vi "WS1050 16 DUT VSA-CV Sweep HD_Cycling_Ver1.1.vi"() -> ()   [LabVIEW 2012]
uses:
  WS_VCAP Driver 024/Source/WSVCAP Shell/Type Defs/WSVCAP SHL I2C DUT Mask Mode Enum.ctl
  <vilib>/Utility/file.llb/Read From Spreadsheet File (DBL).vi
panel:
  out "VISA resource name out":refnum<visa-resource-name>="GPIB0::3::INSTR"
  out "date string":string="5/19/2014"
  out "PS1 Out":refnum<visa-resource-name>
  out "Ke2000 Out":refnum<visa-resource-name>="GPIB0::9::INSTR"
  in  "Tab Control":enum32{"Inst Control", "Data Output", "Graphs"}(tab)
  in  "Bank to Stress":u16(ring) items=["All OFF", "All ON", "Bank_C1", "Bank_C2", "Bank_C3"]
  out "AD7747 Values":string[][](table)
  in  "Lot#":string="4NEMB"
  in  "Wafer#":string="20-EB"
  in  "File Name":string="HD_4NEMB_25_EB_65C_44V_100DC_BRD2_150916_1"
  in  "TMN DC\\CAP Data Log File Path":path=path "C:/WS1050 16 DUT Data"
  in  "SN":string[](array[string])=["1", "2", "3", "4", "5", "6", "7", "8", "9", "10", "11", "12", "13", "14", "15", "16"]
  in  "Test Program":string="WS1050 16 DUT VSA_CV Sweep HD_Cycling Ver1.2"
  out "Current Date":string="8/28/2014"
  out "Current Time":string="0950"
  in  "Start Date":string="4/24/2014"
  in  "Start Time":string="1542"
  in  "Comment":string="VSA CV Sweep"
  in  "OK Button":bool
  in  "Calibration":bool
  in  "Control Setting":bool
  in  "CP Setting":i32(ring) items=["CP OFF", "CP ON", "CP 35V", "CP 40V", "CP 44V", "CP 50V", "DVA OFF", "DVA ON", "Reg1 ON", "Reg1 OFF", "Reg2 ON", "Reg2 OFF", "Reg3 ON", "Reg3 OFF"]
  in  "VDD(V)":dbl=3.3 format="%.3g"
  in  "SPI Clock Rate (Hz)":dbl=1000000.0 caption="Meas Speed" format="%.1p Hz"
  out "AR  Measurent(Hz)":dbl
  in  "PS1 Source":refnum<visa-resource-name>="GPIB0::5::INSTR"
  in  "Ke2000":refnum<visa-resource-name>="GPIB0::9::INSTR"
  out "Simulate FPGA":bool
  out "Online":bool
  in  "Ke2400":refnum<visa-resource-name>="GPIB0::3::INSTR"
  in  "Initialize AD7747":bool
  in  "DUT Mask Mode":T1=enum."All"
  in  "RFFE Slave Address":u8=7 caption="Slave Address" format="0x%02x"
  out "Activity Log":string="05/19/2014 -- 12:24:35.853::WSVCAP::APP::Application Started\n05/19/2014 -- 12:24:37.606::WSVCAP::WSVCAP SHL::WR I2C-REG:0x0A;MASK:0xFFFFFFFFFFFF;C1 DATA:22:22:22:22:22:22:22:22:22:22:22:22:22:22:22:22;C2 DATA:22:22:22:22:22:22:22:22:22:22:22:22:22:22:22:22;C3 DATA:22:22:22:22:22:22:22:22:22:22:22:22:22:22:22:22\r\n05/19/2014 -- 12:24:37.773::WSVCAP::WSVCAP SHL::WR I2C-ST:0,0,4,1\r\n05/19/2014 -- 12:24:37.903::WSVCAP::WSVCAP SHL::RD I2C-BYTES:4;ADD:0x00;MASK:0xFFFFFFFFFFFF\r\n05/19/2014 -- 12:24:38.045::WSVCAP::WSVCAP SHL::RD I2C:C1 DATA:2:2:2:2:2:2:2:2:2:2:2:2:2:2:2:2|A7:A9:AA:82:82:7F:82:81:82:81:83:82:81:82:82:81|46:36:BB:88:44:A3:E9:2B:32:20:ED:25:BB:3D:68:B|2C:6A:EB:A7:22:56:FE:CC:36:82:D7:B0:3B:48:F9:CC;C2 DATA:2:2:2:2:2:2:2:2:2:2:2:2:2:2:2:2|94:94:94:80:80:80:80:80:81:7E:7E:81:80:7E:80:80|47:33:15:82:62:B:E8:1C:D7:C3:7D:41:7C:B7:4C:2A|C4:B4:AE:8:1E:D1:4E:37:11:C0:6F:63:42:9D:63:B5;C3 DATA:2:2:2:2:2:2:2:2:2:2:2:2:2:2:2:2|95:95:95:81:81:7E:81:80:84:7D:80:83:81:7E:7F:80|AB:C4:14:B5:7B:52:DF:C9:79:5D:5F:30:99:31:1E:F4|6E:5C:F7:A8:C3:EB:7B:EF:33:92:89:77:4D:67:75:DD;STATUS:0:0:4:0\r\n05/19/2014 -- 12:24:38.046::WSVCAP::WSVCAP SHL::WR I2C-REG:0x0A;MASK:0xFFFFFFFFFFFF;C1 DATA:22:22:22:22:22:22:22:22:22:22:22:22:22:22:22:22;C2 DATA:22:22:22:22:22:22:22:22:22:22:22:22:22:22:22:22;C3 DATA:22:22:22:22:22:22:22:22:22:22:22:22:22:22:22:22\r\n05/19/2014 -- 12:24:38.089::WSVCAP::WSVCAP SHL::WR I2C-ST:0,0,4,1\r\n05/19/2014 -- 12:24:38.219::WSVCAP::WSVCAP SHL::RD I2C-BYTES:4;ADD:0x00;MASK:0xFFFFFFFFFFFF\r\n05/19/2014 -- 12:24:38.362::WSVCAP::WSVCAP SHL::RD I2C:C1 DATA:2:2:2:2:2:2:2:2:2:2:2:2:2:2:2:2|A7:AB:AA:82:82:82:83:83:82:82:82:82:7F:82:82:81|4B:32:96:83:3E:61:43:17:25:62:AB:4D:A2:40:2E:5|3C:76:2B:B4:EE:E4:A9:1A:AA:A:26:C7:21:2E:87:5B;C2 DATA:2:2:2:2:2:2:2:2:2:2:2:2:2:2:2:2|94:94:94:80:80:80:80:80:80:7F:80:81:80:80:7F:80|4A:32:19:7D:19:6C:79:46:61:7F:4B:B8:A5:30:F3:14|B4:70:A:8C:9C:DC:43:FA:1E:A:C6:21:A:A9:13:F3;C3 DATA:2:2:2:2:2:2:2:2:2:2:2:2:2:2:2:2|95:97:94:81:80:81:82:81:80:7E:81:84:7F:81:80:80|B2:32:D0:A7:9E:4C:AB:D4:EE:D9:F0:82:B7:91:7:FF|C1:91:B6:3D:D8:E:1B:4F:9F:6A:F1:6C:E7:3F:7:BA;STATUS:0:0:4:0\r\n05/19/2014 -- 12:24:38.364::WSVCAP::WSVCAP SHL::WR I2C-REG:0x0A;MASK:0xFFFFFFFFFFFF;C1 DATA:22:22:22:22:22:22:22:22:22:22:22:22:22:22:22:22;C2 DATA:22:22:22:22:22:22:22:22:22:22:22:22:22:22:22:22;C3 DATA:22:22:22:22:22:22:22:22:22:22:22:22:22:22:22:22\r\n05/19/2014 -- 12:24:38.406::WSVCAP::WSVCAP SHL::WR I2C-ST:0,0,4,1\r\n05/19/2014 -- 12:24:38.536::WSVCAP::WSVCAP SHL::RD I2C-BYTES:4;ADD:0x00;MASK:0xFFFFFFFFFFFF\r\n05/19/2014 -- 12:24:38.678::WSVCAP::WSVCAP SHL::RD I2C:C1 DATA:2:2:2:2:2:2:2:2:2:2:2:2:2:2:2:2|A7:A9:AB:82:82:81:82:82:82:82:82:82:82:82:82:81|46:71:4C:87:43:3D:7F:FC:25:4F:8E:54:97:3E:60:8C|AA:F4:1F:B5:CE:43:1F:36:9:87:9C:78:86:5:B6:8E;C2 DATA:2:2:2:2:2:2:2:2:2:2:2:2:2:2:2:2|94:94:94:80:7F:7F:80:80:80:80:80:81:80:80:80:80|49:36:18:7D:6E:C5:E4:3C:81:2E:41:D3:75:71:E3:72|E8:D3:E6:D1:E0:48:AE:D4:54:D:E8:8E:B4:41:68:4;C3 DATA:2:2:2:2:2:2:2:2:2:2:2:2:2:2:2:2|95:95:95:81:7F:7F:81:81:81:81:81:84:81:81:82:81|B3:F5:90:AB:82:69:7B:93:D0:77:E8:D5:E8:8C:84:E8|B9:AC:EE:2B:B6:71:8F:4A:74:31:56:BB:8A:B7:A0:C8;STATUS:0:0:4:0\r\n05/19/2014 -- 12:24:38.681::WSVCAP::WSVCAP SHL::WR I2C-REG:0x0A;MASK:0xFFFFFFFFFFFF;C1 DATA:22:22:22:22:22:22:22:22:22:22:22:22:22:22:22:22;C2 DATA:22:22:22:22:22:22:22:22:22:22:22:22:22:22:22:22;C3 DATA:22:22:22:22:22:22:22:22:22:22:22:22:22:22:22:22\r\n05/19/2014 -- 12:24:38.723::WSVCAP::WSVCAP SHL::WR I2C-ST:0,0,4,1\r\n05/19/2014 -- 12:24:38.854::WSVCAP::WSVCAP SHL::RD I2C-BYTES:4;ADD:0x00;MASK:0xFFFFFFFFFFFF\r\n05/19/2014 -- 12:24:38.996::WSVCAP::WSVCAP SHL::RD I2C:C1 DATA:2:2:2:2:2:2:2:2:2:2:2:2:2:2:2:2|A7:A9:AA:82:82:7F:83:81:82:81:84:82:7F:82:7F:82|43:FB:E:7F:3C:AD:35:35:26:A2:6C:21:4B:3D:8:6|63:9A:E1:F3:95:32:91:42:90:3C:78:1F:5C:D7:5F:D8;C2 DATA:2:2:2:2:2:2:2:2:2:2:2:2:2:2:2:2|94:94:94:80:80:80:80:80:81:80:7E:81:80:7E:7F:80|48:36:18:7F:5E:3D:69:83:DE:AE:A1:9E:31:AE:BB:96|15:A0:44:17:13:FD:CC:C8:6D:B2:EF:A7:C:C7:3B:F;C3 DATA:2:2:2:2:2:2:2:2:2:2:2:2:2:2:2:2|95:96:94:81:81:7E:82:80:84:80:80:84:7F:7E:7D:82|AD:3B:6D:A9:7C:57:9D:F5:7A:96:23:5C:36:2D:ED:5A|CD:46:DB:3B:C7:BD:70:60:33:B8:B:F7:63:A:51:4D;STATUS:0:0:4:0\r\n05/19/2014 -- 12:24:38.998::WSVCAP::WSVCAP SHL::WR I2C-REG:0x0A;MASK:0xFFFFFFFFFFFF;C1 DATA:22:22:22:22:22:22:22:22:22:22:22:22:22:22:22:22;C2 DATA:22:22:22:22:22:22:22:22:22:22:22:22:22:22:22:22;C3 DATA:22:22:22:22:22:22:22:22:22:22:22:22:22:22:22:22\r\n05/19/2014 -- 12:24:39.040::WSVCAP::WSVCAP SHL::WR I2C-ST:0,0,4,1\r\n05/19/2014 -- 12:24:39.170::WSVCAP::WSVCAP SHL::RD I2C-BYTES:4;ADD:0x00;MASK:0xFFFFFFFFFFFF\r\n05/19/2014 -- 12:24:39.311::WSVCAP::WSVCAP SHL::RD I2C:C1 DATA:2:2:2:2:2:2:2:2:2:2:2:2:2:2:2:2|A7:AA:AB:82:82:81:82:81:82:81:82:82:82:82:7F:82|44:F1:90:87:45:44:C8:2C:2C:F1:FC:1B:94:3B:3C:75|4A:49:95:19:99:73:64:3:23:24:F3:A2:5E:7F:C4:B6;C2 DATA:2:2:2:2:2:2:2:2:2:2:2:2:2:2:2:2|94:94:94:80:80:80:80:7F:80:80:7E:80:80:7E:7F:80|4C:36:17:7D:A8:9F:DE:C7:53:6D:8A:F4:41:A5:C6:E0|90:2E:24:C:D9:22:E4:76:3B:40:1D:53:33:B1:3E:4D;C3 DATA:2:2:2:2:2:2:2:2:2:2:2:2:2:2:2:2|95:97:95:81:81:7F:81:80:80:81:7F:82:81:7E:7D:82|AE:2B:A7:AB:CC:CD:A4:38:FD:17:80:F2:92:2D:45:C4|76:E5:D:B9:AD:B5:BA:8D:28:32:9E:42:B7:20:4A:D9;STATUS:0:0:4:0\r\n05/19/2014 -- 12:24:39.313::WSVCAP::WSVCAP SHL::WR I2C-REG:0x0A;MASK:0xFFFFFFFFFFFF;C1 DATA:22:22:22:22:22:22:22:22:22:22:22:22:22:22:22:22;C2 DATA:22:22:22:22:22:22:22:22:22:22:22:22:22:22:22:22;C3 DATA:22:22:22:22:22:22:22:22:22:22:22:22:22:22:22:22\r\n05/19/2014 -- 12:24:39.355::WSVCAP::WSVCAP SHL::WR I2C-ST:0,0,4,1\r\n05/19/2014 -- 12:24:39.486::WSVCAP::WSVCAP SHL::RD I2C-BYTES:4;ADD:0x00;MASK:0xFFFFFFFFFFFF\r\n05/19/2014 -- 12:24:39.628::WSVCAP::WSVCAP SHL::RD I2C:C1 DATA:2:2:2:2:2:2:2:2:2:2:2:2:2:2:2:2|A7:A9:AA:82:82:82:83:82:82:82:82:82:7F:82:7F:82|47:18:E4:87:3E:E7:6:65:25:92:37:38:A8:3E:89:85|7C:A7:7:2B:A3:7A:EC:EF:89:ED:F4:D3:D8:BC:3A:F5;C2 DATA:2:2:2:2:2:2:2:2:2:2:2:2:2:2:2:2|94:94:94:80:7F:80:80:7F:81:80:7E:80:80:80:81:80|49:37:17:80:76:25:6A:F8:DF:55:97:4D:B8:5B:2B:B1|13:E3:9A:3E:1A:2D:4F:B6:DB:E9:61:FA:8B:D6:9:CC;C3 DATA:2:2:2:2:2:2:2:2:2:2:2:2:2:2:2:2|95:95:95:81:7F:80:82:81:84:80:7F:81:80:81:7F:82|AF:93:3B:AF:5B:11:82:E4:7E:C3:2D:72:9:96:D9:A|DB:96:F2:10:5F:64:9A:C6:98:12:27:7D:10:D3:20:D9;STATUS:0:0:4:0\r\n05/19/2014 -- 12:24:40.132::WSVCAP::WSVCAP SHL::CLOSE\r\n"
  in  "C1 Cap DAC":u8=128 caption="B Data In" format="0x%02x"
  in  "C2 Cap DAC":u8=128 caption="B Data In" format="0x%02x"
  in  "C3 Cap DAC":u8=128 caption="B Data In" format="0x%02x"
  out "IDD Brd(uA)":string
  in  "VSA_IDD(A)":dbl=0.1
  in  "Stress Voltage(V)":dbl=10.0
  in  "CP to HD/Cycle":i32(ring)=4 items=["CP HDC 35V", "CP HDC 40.25V", "CP HDC 27.5V", "CP HDC 30.5V", "CP HDC 44V", "CP HDC 50V"]
  in  "Reset PS":bool
  out "STATUS":string="Idle...."
  in  "stop":bool
  out "C1 Min_T0":string[](array[string])
  out "CAP_Value(pF)":string[][](array[string])
  out "C3 Min_T0":string[](array[string])
  out "C2 Min_T0":string[](array[string])
  in  "Abort":bool
  out "error out 2":errorcluster
  in  "Set HD Time \nto Complete(Min)":u64=8100
  out "HD Time\nCompleted(Min)":u64
  out "Verify Test Condition":string[](array[string])
  out "CMin+VCAP":string[][](table)
  out "Previous Time":string="12:20:26 PM"
  out "Running Loops":i32=1
  out "Verify Drivers to Stress":string[](array[string])
  out "Delta CAP_T0(pF)":dbl[][](array[numeric])
  out "Delta CAP_Tc(pF)":dbl[][](array[numeric])
  in  "error in (no error)":errorcluster
  out "error out":errorcluster
  out "CP_IDD(uA)":string
  # "Company:  WiSpry Inc 20 Fairbanks \nSte 198 Irvine CA 92618\n\nAuthor:  Andy V Tran\nCreated:  11/23/2015\nLabVIEW 2012 Pro\nTP:  WS1050 16 DUT VSA_CV Sweep HD_Cycling Ver1.1\nFPGA Version: WS_VCAP Driver 024"
  # "Note:  Ver1.0 is a original version.\n\n1.  Two look up tables, \n      a.  1st is for Stress\n      b.  2nd is for Voltage sweep\n\nVer1.1\n\n1.  No Voltage to CAP Head for initial read point\n\nSet up and Test Sequences:\n\n1.  Calibration with Empty Sockets\n2.  Load Parts\n3.  Set condition to stress (CP Voltage, Drivers to Stress, CP to stress...)\n4.  Set Date/Time to start stressing\n5.  Set TTF to stop stressing (default = 135 hrs)"
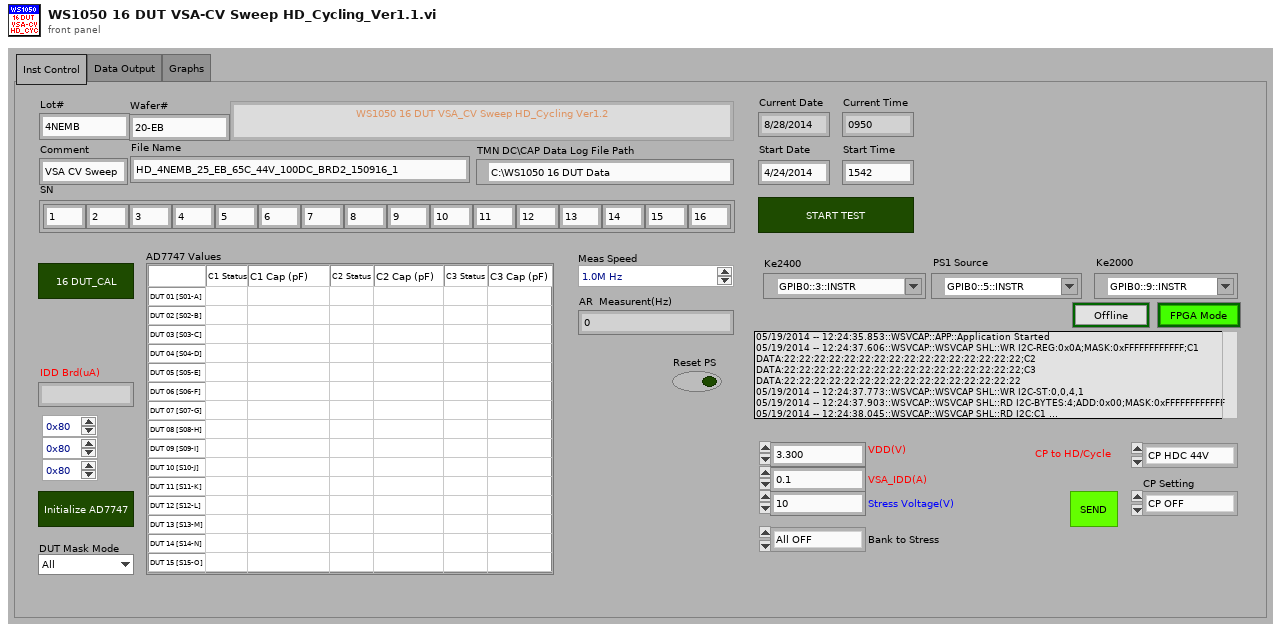
[diagram p1: front panel]
types:
  T1 = typedef "WSVCAP SHL I2C DUT Mask Mode Enum.ctl" = enum16{"Custom", "C1", "C2", "C3", "All"}
  T2 = typedef "WSVCAP SHL Core System Cluster.ctl" = cluster{"Settings":T3, "FPGA Resource":tag, "Online":bool, "I2C Wait Ticks":u32, "SPI Wait Ticks":u32, "RFFE Wait Ticks":u32}
  T3 = typedef "WSVCAP SHL I2C Settings Cluster.ctl" = cluster{"FPGA Resource Name":string, "I2C Slave Address":u8, "I2C Clock Rate (Hz)":dbl, "SPI Clock Rate (Hz)":dbl, "RFFE Slave Address":u8, "RFFE Clock Rate (Hz)":dbl, "Simulate FPGA":bool, "C1 Cap DAC Default":u8, "C2 Cap DAC Default":u8, "C3 Cap DAC Default":u8}
  T4 = enum16{"Idle...", "Voltage 1", "Voltage 2", "Voltage 3"}[]
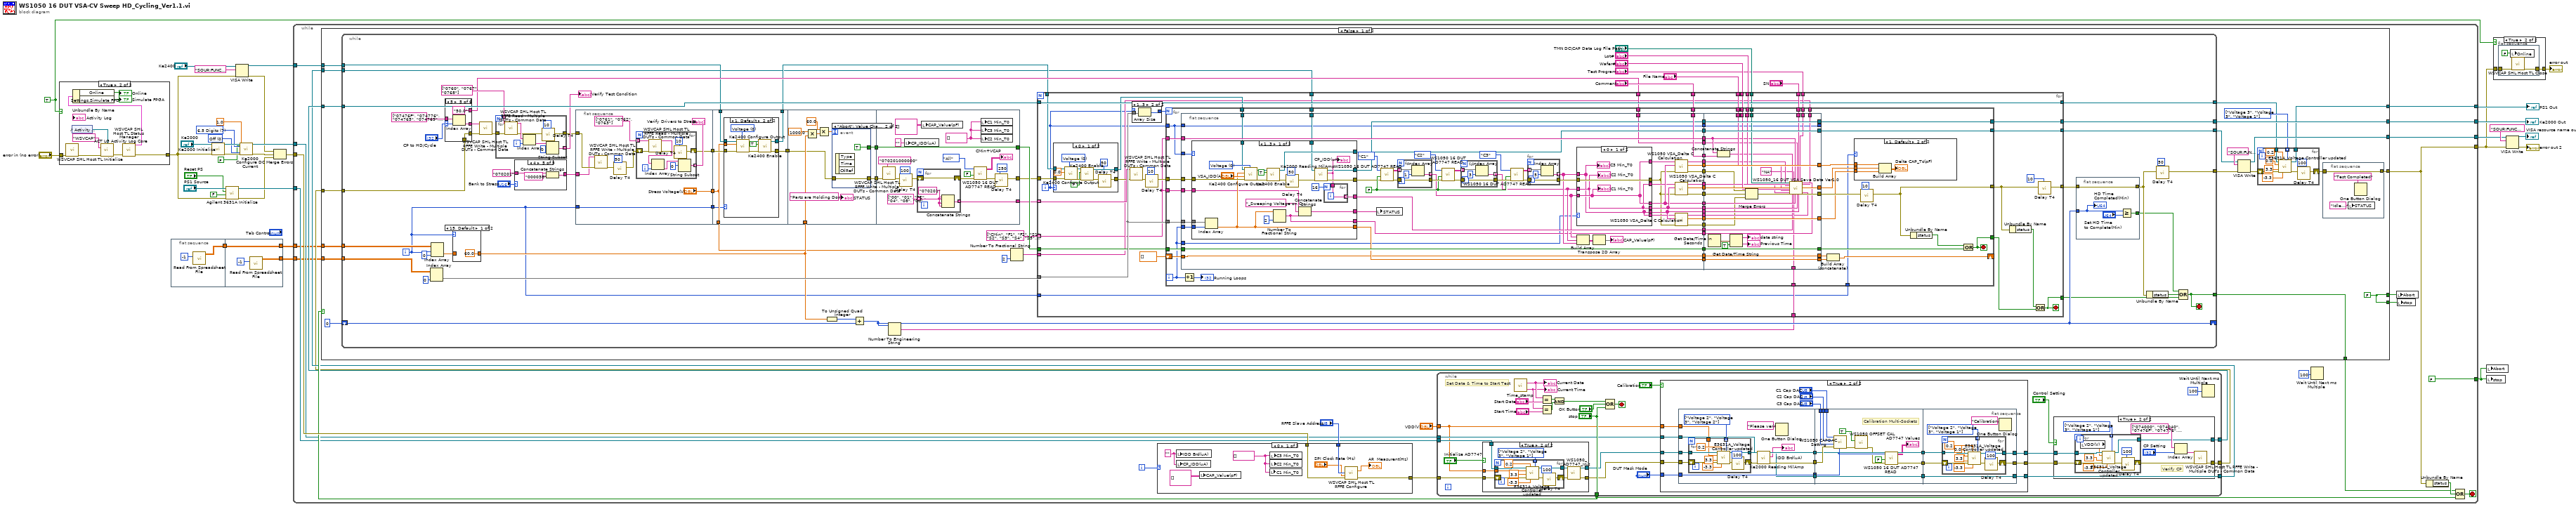
[diagram p0: block diagram]
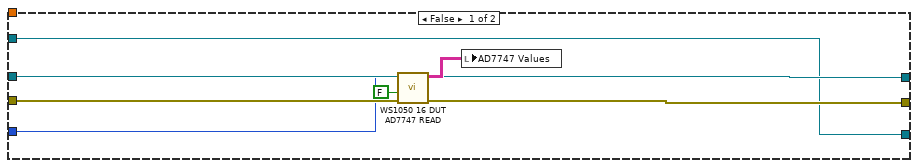
[diagram p7: hidden frame]
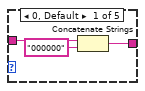
[diagram p8: hidden frame]
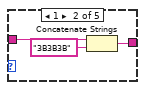
[diagram p9: hidden frame]
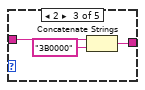
[diagram p10: hidden frame]
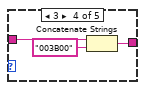
[diagram p11: hidden frame]
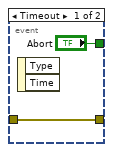
[diagram p14: hidden frame]
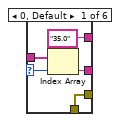
[diagram p15: hidden frame]
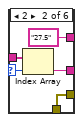
[diagram p16: hidden frame]
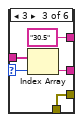
[diagram p17: hidden frame]
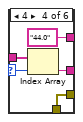
[diagram p18: hidden frame]
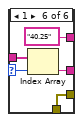
[diagram p19: hidden frame]
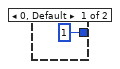
[diagram p20: hidden frame]
diagram:
  w21 = TRUE
  w27 = u16 0 items=["Off", "Moving Filter", "Repeating Filter"] ("Digital Filter (0: Off)")
  w28 = u16 7 items=["3.5 Digits"=4, "4.5 Digits"=5, "5.5 Digits"=6, "6.5 Digits"=7] ("Resolution (7: 6.5 digits)")
  n1 = case shown="True" w21 {
    tunnel: "error in (no error)" -> [w35 w36]
    tunnel: [w35 w43] -> w10
    frame False {
    }
    frame True {
      n2 = call "WSVCAP SHL Host TL Initialize.vi"("error in"=w36) -> ("error out"=w37:errorcluster)  [unwired: 13 in, 1 out]
      n3 = control-ref of="Activity Log"() -> (w39:refnum<vi>)
      n4 = call "ACT LG Activity Log Core.vi"("Display Ref"=w39, "Source"="WSVCAP", "Error In (no error)"=w37) -> ("Error Out"=w38:errorcluster)  [unwired: 11 in, 1 out]
      n5 = call "WSVCAP SHL Host TL Status Manager.vi"("error in"=w38) -> ("System Out"=w44:T2, "error out"=w43:errorcluster)  [unwired: 13 in]
      n6 = Unbundle By Name(w44) -> ("Online"=→"Online":bool, "Settings.Simulate FPGA"=→"Simulate FPGA":bool)
    }
  }
  n7 = flat-sequence {
    tunnel: [w46] -> w5
    tunnel: w5 -> [w49]
    tunnel: [w49] -> w4
    tunnel: [w48] -> w3
    frame #0 {
      n8 = call-poly <vilib>:"Read From Spreadsheet File.vi"("number of rows (all:-1)"=-1) -> ("all rows"=w46:dbl[][])  [unwired: 6 in, 4 out]
    }
    frame #1 {
      n9 = call-poly <vilib>:"Read From Spreadsheet File.vi"("number of rows (all:-1)"=-1) -> ("all rows"=w48:dbl[][])  [unwired: 6 in, 4 out]
    }
  }
  n10 = call "Ke2000 Initialize.vi"("error in (no error)"=w10, "VISA resource name"="Ke2000") -> ("error out"=w29:errorcluster, "VISA resource name out"=w30:refnum<visa-resource-name>)  [unwired: 8 in]
  n11 = call "Agilent 3631A Initialize.vi"("error in (no error)"=w10, "Default"=FALSE ("Reset? (T: Yes)"), "Reset"="Reset PS", "VISA resource name"="PS1 Source") -> ("error out"=w9:errorcluster, "VISA resource name out"=w33:refnum<visa-resource-name>)  [unwired: 6 in]
  n12 = VISA Write(VISA resource name="Ke2400", write buffer="SOUR:FUNC VOLT;VOLT:MODE FIX;RANG 100;LEV 0.0;:SENS:FUNC \"CURR\";CURR:PROT 60E-3;RANG 100E-3;:OUTP ON", error in (no error)=w10) -> (VISA resource name out=w18:refnum<visa-resource-name>, error out=w13:errorcluster)  [unwired: 1 out]
  n13 = call "Ke2000 Configure DC Current.vi"("Resolution (7: 6.5 digits)"=w28, "Digital Filter (0: Off)"=w27, "Auto Range? (T: Auto)"=FALSE, "error in"=w29, "Custom Range (0 A)"=1.0, "VISA resource name"=w30) -> ("error out"=w11:errorcluster, "VISA resource name out"=w25:refnum<visa-resource-name>)  [unwired: 4 in]
  n14 = Merge Errors(w13, w11, w9) -> (w19:errorcluster)
  n15 = while {
    tunnel: w19 -> [w68]
    tunnel: [w57] -> w15
    tunnel: w33 -> [w61]
    tunnel: w25 -> [w62]
    tunnel: [w71] -> w24
    tunnel: [w70] -> w23
    tunnel: w18 -> [w67]
    tunnel: [w66] -> w16
    tunnel: [FALSE] -> w8
    tunnel: w4 -> [w53]
    tunnel: w3 -> [w52]
    i -> [w69]
    stop <- w72 stop-if-true
    n16 = case shown="0" w69 {
      tunnel: w68 -> [w82 w83]
      tunnel: [w81 w83] -> w64
      tunnel: "RFFE Slave Address" -> [w79 _]
      frame 0 {
        w77 = string[] []
        w75 = "" ("uA")
        n17 = local write "IDD Brd(uA)"(w75) -> ()
        n18 = local write "CP_IDD(uA)"(w75) -> ()
        n19 = local write "CAP_Value(pF)"(string[][] []) -> ()
        n20 = local write "C1 Min_T0"(w77) -> ()
        n21 = local write "C3 Min_T0"(w77) -> ()
        n22 = local write "C2 Min_T0"(w77) -> ()
        n23 = call "WSVCAP SHL Host TL RFFE Configure.vi"("RFFE Slave Address"=w79, "Clock Rate (Hz)"="SPI Clock Rate (Hz)", "error in"=w82) -> ("Actual Rate (Hz)"=→"AR  Measurent(Hz)":dbl, "error out"=w81:errorcluster)  [unwired: 11 in]
      }
      frame 1, Default {
      }
    }
    n24 = while {
      tunnel: ["stop"] -> w65
      tunnel: w64 -> [w95]
      tunnel: [w87] -> w58
      tunnel: w61 -> [w93]
      tunnel: w62 -> [w89]
      tunnel: [w90] -> w60
      tunnel: [w88] -> w59
      tunnel: "VDD(V)" -> [w85]
      stop <- w102 stop-if-true
      # "Set Date & Time to Start Test"
      n25 = case shown="True" "Initialize AD7747" {
        tunnel: w95 -> [w111 w117]
        tunnel: [w111 w113] -> w94
        tunnel: w93 -> [w110 w115]
        tunnel: [w110 w114] -> w92
        tunnel: w85 -> [_ w112]
        frame False {
        }
        frame True {
          w118 = T4 [enum."Voltage 2", enum."Voltage 3", enum."Voltage 1"] items=["Idle...", "Voltage 1", "Voltage 2", "Voltage 3"]
          n26 = for {
            tunnel: w115 -> [w128]
            tunnel: w118 -> [w126] mode=indexing
            tunnel: [w125] -> w114
            shift-right: [w122] -> w116
            shift-left: w117 -> [w129]
            tunnel: w112 -> [w120]
            n27 = call "E3631A_Voltage Controller updated.vi"("VISA resource name"=w128, "I_VDD(A)"=0.2, "Channel Controller"=w126, "Voltage 1"=w120, "Voltage 2"=3.3, "error in (no error)"=w129, "Voltage 3"=-3.3) -> ("VISA resource name out"=w125:refnum<visa-resource-name>, "error out"=w121:errorcluster)  [unwired: 7 in]
            n28 = call "Delay T4.vi"("milliseconds to wait"=u32 100, "error in (no error)"=w121) -> ("error out"=w122:errorcluster)  [unwired: 9 in]
          }
          n29 = call "WS1050_AD7747_Init.vi"("error in"=w116) -> ("error out"=w113:errorcluster)  [unwired: 10 in]
        }
      }
      n30 = call "Time_stamp.vi"() -> ("date/time string"=w107:string, "date string"=w109:string)  [unwired: 2 in]
      "Current Date" <- w109
      "Current Time" <- w107
      n31 = Equal?(x=w109, y="Start Date") -> (x = y?=w105:bool)
      n32 = Equal?(x=w107, y="Start Time") -> (x = y?=w104:bool)
      n33 = And(x=w105, y=w104) -> (x .and. y?=w101:bool)
      n34 = Compound Arithmetic op=OR(w101, "OK Button", "stop") -> (w102:bool)
      n35 = case shown="True" "Calibration" {
        tunnel: w94 -> [w156 w175]
        tunnel: [w155 w172] -> w86
        tunnel: w92 -> [w154 w171]
        tunnel: "DUT Mask Mode" -> [w153 w167]
        tunnel: [w154 w166] -> w91
        tunnel: w89 -> [w152 w162]
        tunnel: [w152 w159] -> w88
        tunnel: w85 -> [_ w158]
        frame False {
          n36 = call "WS1050 16 DUT AD7747 READ.vi"("error in"=w156, "Log (T)"=FALSE, "DUT Mask Mode (All)"=w153) -> ("error out"=w155:errorcluster, "AD7747 Values"=w157:string[][])  [unwired: 7 in]
          n37 = local write "AD7747 Values"(w157) -> ()
        }
        frame True {
          n38 = flat-sequence {
            tunnel: w175 -> [w185]
            tunnel: [w180] -> w174
            tunnel: w171 -> [w184]
            tunnel: [w183] -> w170
            tunnel: w167 -> [w182]
            tunnel: [w182] -> w168
            tunnel: w162 -> [w178]
            tunnel: [w177] -> w161
            tunnel: w158 -> [w176]
            tunnel: w174 -> [w211]
            tunnel: [w210] -> w173
            tunnel: w170 -> [w209]
            tunnel: [w209] -> w169
            tunnel: w168 -> [w208]
            tunnel: "C1 Cap DAC" -> [w204]
            tunnel: "C2 Cap DAC" -> [w203]
            tunnel: "C3 Cap DAC" -> [w202]
            tunnel: w161 -> [w201]
            tunnel: [w201] -> w160
            tunnel: w173 -> [w214]
            tunnel: [w217] -> w172
            tunnel: w169 -> [w216]
            tunnel: [w213] -> w166
            tunnel: w160 -> [w212]
            tunnel: [w212] -> w159
            frame #0 {
              w186 = T4 [enum."Voltage 2", enum."Voltage 3", enum."Voltage 2"] items=["Idle...", "Voltage 1", "Voltage 2", "Voltage 3"]
              n39 = for {
                tunnel: w184 -> [w197]
                tunnel: w186 -> [w194] mode=indexing
                tunnel: [w193] -> w183
                shift-right: [w191] -> w179
                shift-left: w185 -> [w198]
                tunnel: w176 -> [w188]
                n40 = call "E3631A_Voltage Controller updated.vi"("VISA resource name"=w197, "I_VDD(A)"=0.2, "Channel Controller"=w194, "Voltage 1"=w188, "Voltage 2"=3.3, "error in (no error)"=w198, "Voltage 3"=-3.3) -> ("VISA resource name out"=w193:refnum<visa-resource-name>, "error out"=w190:errorcluster)  [unwired: 7 in]
                n41 = call "Delay T4.vi"("milliseconds to wait"=u32 100, "error in (no error)"=w190) -> ("error out"=w191:errorcluster)  [unwired: 9 in]
              }
              n42 = call "Ke2000 Reading MilAmp.vi"("error in (no error)"=w179, "VISA resource name"=w178) -> ("error out"=w180:errorcluster, "uA"=→"IDD Brd(uA)":string, "VISA resource name out"=w177:refnum<visa-resource-name>)  [unwired: 7 in]
              n43 = One Button Dialog(message="Please verify all sockets should be empty...") -> ()  [unwired: 1 in, 1 out]
            }
            frame #1 {
              # "Calibration Multi-Sockets"
              n44 = call "WS1050 CAPDAC Setting.vi"("DUT Mask Mode (All)"=w208, "error in"=w211, "C3 Cap DAC"=w202, "C2 Cap DAC"=w203, "C1 Cap DAC"=w204) -> ("error out"=w206:errorcluster)  [unwired: 5 in, 1 out]
              n45 = call "WS1050 OFFSET CAL.vi"("error in"=w206, "OFFSET CAL"=TRUE ("Read?")) -> ("error out"=w205:errorcluster)  [unwired: 8 in, 1 out]
              n46 = call "WS1050 16 DUT AD7747 READ.vi"("error in"=w205, "Log (T)"=FALSE, "DUT Mask Mode (All)"=w208) -> ("error out"=w210:errorcluster, "AD7747 Values"=→"AD7747 Values":string[][])  [unwired: 7 in]
            }
            frame #2 {
              w215 = T4 [enum."Voltage 2", enum."Voltage 3", enum."Voltage 1"] items=["Idle...", "Voltage 1", "Voltage 2", "Voltage 3"]
              n47 = for {
                tunnel: w216 -> [w229]
                tunnel: w215 -> [w225] mode=indexing
                tunnel: [w224] -> w213
                shift-right: [w220] -> w217
                shift-left: w214 -> [w226]
                n48 = call "E3631A_Voltage Controller updated.vi"("VISA resource name"=w229, "I_VDD(A)"=0.2, "Channel Controller"=w225, "Voltage 1"=0.0, "Voltage 2"=3.3, "error in (no error)"=w226, "Voltage 3"=-3.3) -> ("VISA resource name out"=w224:refnum<visa-resource-name>, "error out"=w219:errorcluster)  [unwired: 7 in]
                n49 = call "Delay T4.vi"("milliseconds to wait"=u32 100, "error in (no error)"=w219) -> ("error out"=w220:errorcluster)  [unwired: 9 in]
              }
              n50 = One Button Dialog(message="Calibration Completed....") -> ()  [unwired: 1 in, 1 out]
            }
          }
        }
      }
      n51 = case shown="True" "Control Setting" {
        tunnel: [w130 w133] -> w87
        tunnel: w91 -> [w131 w136]
        tunnel: [w131 w134] -> w90
        tunnel: w86 -> [w130 w132]
        frame False {
        }
        frame True {
          w137 = T4 [enum."Voltage 2", enum."Voltage 3", enum."Voltage 1"] items=["Idle...", "Voltage 1", "Voltage 2", "Voltage 3"]
          # "Verify CP"
          n52 = for {
            tunnel: w136 -> [w149]
            tunnel: w137 -> [w146] mode=indexing
            shift-right: [w143] -> w135
            shift-left: w132 -> [w150]
            tunnel: [w141] -> w134
            n53 = local read "VDD(V)"() -> (w145:dbl)
            n54 = call "E3631A_Voltage Controller updated.vi"("VISA resource name"=w149, "Channel Controller"=w146, "Voltage 1"=w145, "Voltage 2"=3.3, "error in (no error)"=w150, "Voltage 3"=-3.3) -> ("VISA resource name out"=w141:refnum<visa-resource-name>, "error out"=w144:errorcluster)  [unwired: 8 in]
            n55 = call "Delay T4.vi"("milliseconds to wait"=u32 100, "error in (no error)"=w144) -> ("error out"=w143:errorcluster)  [unwired: 9 in]
          }
          n56 = Index Array(array=string[] ["074000", "074040", "07476F", "074776", "07477B", "07477C", "074820", "074800", "07413B", "074100", "07423B", "074200", "07433B", "074300"], index="CP Setting") -> (element=w138:string)
          n57 = call "WSVCAP SHL Host TL RFFE Write - Multiple DUTs - Common Data.vi"("Data Out"=w138, "error in"=w135) -> ("error out"=w133:errorcluster)  [unwired: 13 in]
        }
      }
      n58 = Wait Until Next ms Multiple(millisecond multiple=u32 100) -> ()  [unwired: 1 out]
    }
    n59 = case shown="False" w65 {
      tunnel: w58 -> [w246 w734]
      tunnel: [w230 w734] -> w57
      tunnel: w60 -> [w244 w732]
      tunnel: w59 -> [w247 w733]
      tunnel: [w243 w733] -> w71
      tunnel: [w234 w732] -> w70
      tunnel: w67 -> [w249 w731]
      tunnel: [w245 w731] -> w66
      tunnel: [w242 w730] -> w55
      tunnel: [w242 w730] -> w54
      tunnel: w53 -> [w240 _]
      tunnel: w52 -> [w238 _]
      tunnel: [w233 w730] -> w50
      frame False {
        w237 = T4 [enum."Voltage 3", enum."Voltage 3", enum."Voltage 1"] items=["Idle...", "Voltage 1", "Voltage 2", "Voltage 3"]
        w242 = FALSE
        n60 = while {
          tunnel: w249 -> [w277]
          tunnel: w247 -> [w273]
          tunnel: w246 -> [w268]
          tunnel: w244 -> [w315]
          tunnel: [w314] -> w243
          tunnel: [w313] -> w235
          tunnel: [w312] -> w241
          tunnel: [w311] -> w232
          tunnel: w240 -> [w303]
          shift-right: [w294] -> _
          shift-left: u64 0 ("disabled index (col)") -> [w300]
          tunnel: w238 -> [w292]
          tunnel: [w267] -> w233
          i -> [w265]
          stop <- w267 stop-if-true
          n61 = Index Array(array=w292, index (col)=0 ("disabled index (col)")) -> (element=w291:dbl[])  [unwired: 1 in]
          n62 = Index Array(array=w303, index (row)=w265, index (col)=0 ("disabled index (col)")) -> (element=w281:dbl)
          n63 = case shown="5" "CP to HD/Cycle" {
            selector: "CP to HD/Cycle" -> [w427 w432 w437 w442 w447 w451]
            tunnel: string[] ["07476F", "074776", "074765", "074769", "07477B", "07477C"] -> [w428 w433 w438 w443 w448 w453]
            tunnel: [w426 w431 w436 w441 w446 w452] -> w308
            tunnel: ["35.0" ("Data Out") "27.5" ("Data Out") "30.5" ("Data Out") "44.0" ("Data Out") "50.0" ("Data Out") "40.25" ("Data Out")] -> w287
            tunnel: [w424 w429 w434 w439 w444 w449] -> w307
            tunnel: w268 -> [w424 w429 w434 w439 w444 w449]
            frame 0, Default {
              n64 = Index Array(array=w428, index=w427) -> (element=w426:string)
            }
            frame 2 {
              n65 = Index Array(array=w433, index=w432) -> (element=w431:string)
            }
            frame 3 {
              n66 = Index Array(array=w438, index=w437) -> (element=w436:string)
            }
            frame 4 {
              n67 = Index Array(array=w443, index=w442) -> (element=w441:string)
            }
            frame 5 {
              n68 = Index Array(array=w448, index=w447) -> (element=w446:string)
            }
            frame 1 {
              n69 = Index Array(array=w453, index=w451) -> (element=w452:string)
            }
          }
          n70 = case shown="15, Default" w265 {
            tunnel: w281 -> [_ w337]
            tunnel: [60.0 w337] -> w280
            frame 15, Default {
            }
            frame 0..14 {
            }
          }
          n71 = call "WSVCAP SHL Host TL RFFE Write - Multiple DUTs - Common Data.vi"("Data Out"=w308, "error in"=w307) -> ("error out"=w305:errorcluster)  [unwired: 13 in]
          n72 = for {
            tunnel: string[] ["0760", "0767", "0768"] -> [w423] mode=indexing
            tunnel: [w419] -> w304 mode=indexing
            tunnel: w305 -> [w417]
            tunnel: [w415] -> w298
            i -> [w422]
            n73 = call "WSVCAP SHL Host TL RFFE Read - Multiple DUTs - Common Data.vi"("Data Out"=w423, "error in"=w417) -> ("RFFE Data In"=w421:string[], "error out"=w414:errorcluster)  [unwired: 12 in]
            n74 = Index Array(array=w421, index=w422) -> (element=w418:string)
            n75 = call "Delay T4.vi"("milliseconds to wait"=u32 10, "error in (no error)"=w414) -> ("error out"=w415:errorcluster)  [unwired: 9 in]
            n76 = String Subset(string=w418, offset (0)=0) -> (substring=w419:string)  [unwired: 1 in]
          }
          "Verify Test Condition" <- w304
          n77 = case shown="4" "Bank to Stress" {
            tunnel: "070201" -> [w323 w325 w328 w331 w334]
            tunnel: [w321 w324 w327 w330 w333] -> w262
            frame 0, Default {
              n78 = Concatenate Strings(w323, "000000" ("string")) -> (w321:string)
            }
            frame 1 {
              n79 = Concatenate Strings(w325, "3B3B3B" ("string")) -> (w324:string)
            }
            frame 2 {
              n80 = Concatenate Strings(w328, "3B0000" ("string")) -> (w327:string)
            }
            frame 3 {
              n81 = Concatenate Strings(w331, "003B00" ("string")) -> (w330:string)
            }
            frame 4 {
              n82 = Concatenate Strings(w334, "00003B" ("string")) -> (w333:string)
            }
          }
          n83 = flat-sequence {
            tunnel: [w345] -> w279
            tunnel: w298 -> [w351]
            tunnel: ["Stress Voltage(V)"] -> w276
            tunnel: w265 -> [w343]
            tunnel: [w343] -> w266
            tunnel: w262 -> [w342]
            tunnel: w279 -> [w366]
            tunnel: [w367] -> w278
            tunnel: w277 -> [w365]
            tunnel: [w364] -> w275
            tunnel: w276 -> [w363]
            tunnel: [w363] -> w271
            tunnel: w266 -> [w362]
            tunnel: w278 -> [w381]
            tunnel: w280 -> [w383]
            tunnel: [w382] -> w286
            tunnel: [w380] -> w285
            tunnel: [w396] -> w284
            tunnel: [w409] -> w290
            tunnel: w286 -> [w409]
            tunnel: w285 -> [w405]
            tunnel: [w407] -> w274
            frame #0 {
              n84 = call "WSVCAP SHL Host TL RFFE Write - Multiple DUTs - Common Data.vi"("Data Out"=w342, "error in"=w351) -> ("error out"=w350:errorcluster)  [unwired: 13 in]
              n85 = call "Delay T4.vi"("milliseconds to wait"=u32 50, "error in (no error)"=w350) -> ("error out"=w347:errorcluster)  [unwired: 9 in]
              n86 = for {
                tunnel: string[] ["0761", "0762", "0763"] -> [w361] mode=indexing
                tunnel: [w357] -> w346 mode=indexing
                shift-right: [w354] -> w345
                shift-left: w347 -> [w360]
                i -> [w359]
                n87 = call "WSVCAP SHL Host TL RFFE Read - Multiple DUTs - Common Data.vi"("Data Out"=w361, "error in"=w360) -> ("RFFE Data In"=w356:string[], "error out"=w353:errorcluster)  [unwired: 12 in]
                n88 = Index Array(array=w356, index=w359) -> (element=w355:string)
                n89 = call "Delay T4.vi"("milliseconds to wait"=u32 10, "error in (no error)"=w353) -> ("error out"=w354:errorcluster)  [unwired: 9 in]
                n90 = String Subset(string=w355, offset (0)=0) -> (substring=w357:string)  [unwired: 1 in]
              }
              "Verify Drivers to Stress" <- w346
            }
            frame #1 {
              n91 = case shown="1, Default" w362 {
                tunnel: [w368 w375] -> w367
                tunnel: w366 -> [w368 w374]
                tunnel: w365 -> [w369 w373]
                tunnel: [w369 w372] -> w364
                tunnel: w363 -> [_ w370]
                frame 0 {
                }
                frame 1, Default {
                  w371 = u16 0 items=["Voltage", "Current"] ("Source Mode  (0: Voltage)")
                  n92 = call "Ke2400 Configure Output.vi"("Source Mode  (0: Voltage)"=w371, "error in (no error)"=w374, "Output Level (0)"=w370, "VISA resource name"=w373) -> ("error out"=w378:errorcluster, "VISA resource name out"=w376:refnum<visa-resource-name>)  [unwired: 6 in]
                  n93 = call "Ke2400 Enable.vi"("error in (no error)"=w378, "ON/OFF"=TRUE ("Enable Output (T: Enable)"), "VISA resource name"=w376) -> ("error out"=w375:errorcluster, "VISA resource name out"=w372:refnum<visa-resource-name>)  [unwired: 7 in]
                }
              }
            }
            frame #2 {
              n94 = Multiply(x=1000.0, y=w383) -> (x*y=w386:dbl)
              n95 = Multiply(x=60.0, y=w386) -> (x*y=w387:dbl)
              n96 = event shown="[1] \"Abort\": Value Change" {
                selector: _ -> [_ _]
                dyn-events: _ -> [_ _]
                timeout: w387 -> [_ _]
                tunnel: ["Abort" TRUE ("Abort")] -> w382
                tunnel: w381 -> [w388 w390]
                tunnel: [w388 w390] -> w380
                event Timeout {
                  n97 = event-data() -> ()  [unwired: 1 in, 2 out]
                }
                event "Abort": Value Change {
                  n98 = event-data() -> ()  [unwired: 1 in, 3 out]
                }
              }
              "STATUS" <- "Parts are Holding Down...." ("STATUS")
            }
            frame #3 {
              w403 = string[] [] ("CP Current(uA)")
              n99 = call "WSVCAP SHL Host TL RFFE Write - Multiple DUTs - Common Data.vi"("Data Out"="070201000000", "error in"=w405) -> ("error out"=w399:errorcluster)  [unwired: 13 in]
              n100 = call "Delay T4.vi"("milliseconds to wait"=u32 100, "error in (no error)"=w399) -> ("error out"=w400:errorcluster)  [unwired: 9 in]
              n101 = local write "CP_IDD(uA)"("" ("CP_IDD(uA)")) -> ()
              n102 = for {
                tunnel: string[] ["00", "01", "02", "04", "08", "0C", "10", "14", "18", "1C", "20", "24", "28", "2C", "30", "34", "38", "3B", "00"] -> [w412] mode=indexing
                tunnel: [w411] -> w407 mode=indexing
                shift-right: [w410] -> w404
                shift-left: w400 -> [w410]
                n103 = Concatenate Strings("070201" ("string"), w412, w412, w412) -> (w411:string)
              }
              n104 = local write "CAP_Value(pF)"(string[][] [] ("VSA_Value(pF)")) -> ()
              n105 = call "WS1050 16 DUT AD7747 READ.vi"("error in"=w404, "Log (T)"=FALSE, "DUT Mask Mode (All)"=WSVCAP_SHL_I2C_DUT_Mask_Mode_Enum."All") -> ("error out"=w395:errorcluster, "AD7747 Values"=→"CMin+VCAP":string[][])  [unwired: 7 in]
              n106 = local write "C1 Min_T0"(w403) -> ()
              n107 = local write "C3 Min_T0"(w403) -> ()
              n108 = local write "C2 Min_T0"(w403) -> ()
              n109 = call "Delay T4.vi"("milliseconds to wait"=u32 250, "error in (no error)"=w395) -> ("error out"=w396:errorcluster)  [unwired: 9 in]
            }
          }
          n110 = To Unsigned Quad Integer(1:w280) -> (0:w301:u64)
          n111 = Add(x=w301, y=w300) -> (x+y=w294:u64)
          n112 = Number To Engineering String(4:w294) -> (0:w288:string)  [unwired: 3 in]
          n113 = Number To Fractional String(number=w271, precision (6)=i16 2) -> (F-format string=w270:string)  [unwired: 2 in]
          n114 = for {
            tunnel: w284 -> [w464]
            tunnel: [w488] -> w312
            tunnel: [w471] -> w297
            tunnel: "Comment" -> [w486]
            tunnel: "Lot#" -> [w485]
            tunnel: "Wafer#" -> [w484]
            tunnel: "SN" -> [w483]
            tunnel: "File Name" -> [w482]
            tunnel: [w481] -> w313
            tunnel: w315 -> [w481]
            tunnel: [w480] -> w314
            tunnel: w291 -> [w477]
            tunnel: w290 -> [w476]
            tunnel: [w473] -> w289
            tunnel: w288 -> [w455]
            tunnel: w287 -> [w472]
            tunnel: "TMN DC\\CAP Data Log File Path" -> [w469]
            tunnel: "Test Program" -> [w468]
            tunnel: w275 -> [w462]
            tunnel: w274 -> [w466] mode=indexing
            tunnel: w273 -> [w461]
            tunnel: string[] ["CMin", "F1", "F2", "S1", "S2", "S3", "S4", "S5", "S6", "S7", "S8", "S9", "S10", "S11", "S12", "S13", "S14", "S14F12", "All OFF"] -> [w459] mode=indexing
            tunnel: w270 -> [w460]
            tunnel: w265 -> [w454]
            i -> [w456]
            stop <- w473 stop-if-true
            n115 = case shown="0" w456 {
              tunnel: [w494 w504] -> w465
              tunnel: w464 -> [w501 w504]
              tunnel: [w500 w503] -> w463
              tunnel: w462 -> [w499 w503]
              frame 0 {
                w497 = u16 0 items=["Voltage", "Current"] ("Source Mode  (0: Voltage)")
                n116 = call "Ke2400 Configure Output.vi"("Source Mode  (0: Voltage)"=w497, "error in (no error)"=w501, "Output Level (0)"=0.0, "VISA resource name"=w499) -> ("error out"=w502:errorcluster, "VISA resource name out"=w495:refnum<visa-resource-name>)  [unwired: 6 in]
                n117 = call "Ke2400 Enable.vi"("error in (no error)"=w502, "ON/OFF"=TRUE ("Enable Output (T: Enable)"), "VISA resource name"=w495) -> ("error out"=w493:errorcluster, "VISA resource name out"=w500:refnum<visa-resource-name>)  [unwired: 7 in]
                n118 = call "Delay T4.vi"("milliseconds to wait"=u32 50, "error in (no error)"=w493) -> ("error out"=w494:errorcluster)  [unwired: 9 in]
              }
              frame 1, Default {
              }
            }
            n119 = call "WSVCAP SHL Host TL RFFE Write - Multiple DUTs - Common Data.vi"("Data Out"=w466, "error in"=w465) -> ("error out"=w467:errorcluster)  [unwired: 13 in]
            n120 = case shown="1..3" w456 {
              tunnel: [1 w491] -> w487
              tunnel: w477 -> [_ w490]
              frame 0, Default {
              }
              frame 1..3 {
                n121 = Array Size(array=w490) -> (size(s)=w491:i32)
              }
            }
            n122 = call "Delay T4.vi"("milliseconds to wait"=u32 10, "error in (no error)"=w467) -> ("error out"=w479:errorcluster)  [unwired: 9 in]
            n123 = for {
              N: w487 -> [_]
              tunnel: w477 -> [w563]
              tunnel: w469 -> [w552]
              tunnel: [w561] -> w458
              tunnel: w479 -> [w560]
              tunnel: [w556] -> w488
              tunnel: w486 -> [w539]
              tunnel: w485 -> [w546]
              tunnel: w484 -> [w545]
              tunnel: w483 -> [w544]
              tunnel: w482 -> [w543]
              tunnel: w459 -> [w542]
              tunnel: [w537] -> w480
              tunnel: w463 -> [w529]
              tunnel: w476 -> [w528]
              tunnel: [w525] -> w474
              tunnel: w472 -> [w523]
              tunnel: w468 -> [w522]
              tunnel: w461 -> [w521]
              tunnel: w460 -> [w520]
              tunnel: w459 -> [w519]
              shift-right: [w513] -> _
              shift-left: dbl[] [] -> [w516]
              tunnel: w456 -> [w511]
              tunnel: w455 -> [w510]
              tunnel: w454 -> [w505]
              i -> [w509]
              stop <- w525 stop-if-true
              n124 = flat-sequence {
                tunnel: w563 -> [w625]
                tunnel: w509 -> [w624]
                tunnel: w560 -> [w626]
                tunnel: [w591] -> w557
                tunnel: [w605] -> w555
                tunnel: [w606] -> w554
                tunnel: [w607] -> w553
                tunnel: [w576] -> w551
                tunnel: [w608] -> w550
                tunnel: [w604] -> w549
                tunnel: [w603] -> w548
                tunnel: [w602] -> w547
                tunnel: w542 -> [w601]
                tunnel: [w601] -> w541
                tunnel: [w600] -> w540
                tunnel: w539 -> [w600]
                tunnel: [w599] -> w538
                tunnel: [w598] -> w535
                tunnel: [w597] -> w534
                tunnel: [w596] -> w533
                tunnel: [w586] -> w532
                tunnel: [w585] -> w531
                tunnel: [w584] -> w530
                tunnel: w529 -> [w583]
                tunnel: w528 -> [w582]
                tunnel: [w582] -> w527
                tunnel: [w581] -> w524
                tunnel: w523 -> [w581]
                tunnel: w511 -> [w579]
                tunnel: w521 -> [w578]
                tunnel: w519 -> [w577]
                tunnel: [w575] -> w518
                tunnel: w516 -> [w574]
                tunnel: [w574] -> w515
                tunnel: w511 -> [w573]
                tunnel: [w573] -> w512
                tunnel: w509 -> [w572]
                tunnel: [w724] -> w558
                tunnel: [w726] -> w556
                tunnel: [w725] -> w537
                tunnel: [w723] -> w508
                tunnel: [w722] -> w507
                tunnel: [w721] -> w506
                tunnel: w533 -> [w723]
                tunnel: w534 -> [w722]
                tunnel: w535 -> [w721]
                tunnel: w538 -> [w725]
                tunnel: w540 -> [w708]
                tunnel: w541 -> [w695]
                tunnel: w547 -> [w709]
                tunnel: w548 -> [w710]
                tunnel: w549 -> [w711]
                tunnel: w543 -> [w712]
                tunnel: w550 -> [w713]
                tunnel: w551 -> [w706]
                tunnel: w544 -> [w714]
                tunnel: w545 -> [w715]
                tunnel: w546 -> [w716]
                tunnel: w552 -> [w717]
                tunnel: w553 -> [w718]
                tunnel: w554 -> [w719]
                tunnel: w555 -> [w720]
                tunnel: w557 -> [w726]
                tunnel: w532 -> [w699]
                tunnel: w531 -> [w700]
                tunnel: w530 -> [w698]
                tunnel: w527 -> [w696]
                tunnel: [w696] -> w526
                tunnel: w524 -> [w694]
                tunnel: w522 -> [w693]
                tunnel: w520 -> [w692]
                tunnel: w518 -> [w691]
                tunnel: [w691] -> w517
                tunnel: w515 -> [w690]
                tunnel: [w690] -> w514
                tunnel: w512 -> [w689]
                tunnel: [w689] -> _
                tunnel: w510 -> [w688]
                frame #0 {
                  w612 = FALSE ("Log (T)")
                  n125 = case shown="1..3" w579 {
                    tunnel: w626 -> [w651 w658]
                    tunnel: w625 -> [w650 _]
                    tunnel: w624 -> [w649 _]
                    tunnel: [w640 w658] -> w609
                    tunnel: [w638 w661] -> w608
                    tunnel: [w637 w656] -> w599
                    tunnel: [w632 0.0] -> w575
                    tunnel: [w636 w657] -> w591
                    tunnel: w583 -> [w634 w657]
                    tunnel: [w630 "0"] -> w576
                    tunnel: [w629 w653] -> w580
                    tunnel: w578 -> [w628 w656]
                    tunnel: w577 -> [w627 w654]
                    frame 1..3 {
                      w643 = u16 0 items=["Voltage", "Current"] ("Source Mode  (0: Voltage)")
                      n126 = Index Array(array=w650, index=w649) -> (element=w632:dbl)
                      n127 = call "Ke2400 Configure Output.vi"("Source Mode  (0: Voltage)"=w643, "error in (no error)"=w651, "Compliance  Level (0.1)"="VSA_IDD(A)", "Output Level (0)"=w632, "VISA resource name"=w634) -> ("error out"=w647:errorcluster, "VISA resource name out"=w645:refnum<visa-resource-name>)  [unwired: 5 in]
                      n128 = call "Ke2400 Enable.vi"("error in (no error)"=w647, "ON/OFF"=TRUE ("Enable Output (T: Enable)"), "VISA resource name"=w645) -> ("error out"=w648:errorcluster, "VISA resource name out"=w636:refnum<visa-resource-name>)  [unwired: 7 in]
                      n129 = Number To Fractional String(number=w632, precision (6)=i16 2) -> (F-format string=w630:string)  [unwired: 2 in]
                      n130 = call "Delay T4.vi"("milliseconds to wait"=u32 50, "error in (no error)"=w648) -> ("error out"=w635:errorcluster)  [unwired: 9 in]
                      n131 = Concatenate Strings(w627, "_Sweeping Voltage on CAP Head... ", w630) -> (w629:string)
                      n132 = call "Ke2000 Reading MilAmp.vi"("error in (no error)"=w635, "VISA resource name"=w628) -> ("error out"=w640:errorcluster, "uA"=w639:string, "VISA resource name out"=w637:refnum<visa-resource-name>)  [unwired: 7 in]
                      "CP_IDD(uA)" <- w639
                      n133 = for {
                        N: 16 -> [_]
                        tunnel: w639 -> [w652]
                        tunnel: [w652] -> w638 mode=indexing
                      }
                    }
                    frame 0, Default {
                      n134 = Concatenate Strings(w654, "_No Sweeping Voltage on CAP Head... ") -> (w653:string)
                      n135 = for {
                        N: 16 -> [_]
                        tunnel: "0" ("uA") -> [w664]
                        tunnel: [w664] -> w661 mode=indexing
                      }
                    }
                  }
                  n136 = local write "STATUS"(w580) -> ()
                  n137 = call "WS1050 16 DUT AD7747 READ.vi"("error in"=w609, "Log (T)"=w612, "DUT Mask Mode (All)"=WSVCAP_SHL_I2C_DUT_Mask_Mode_Enum."C1") -> ("error out"=w621:errorcluster, "AD7747 Values"=w623:string[][])  [unwired: 7 in]
                  n138 = for {
                    tunnel: w623 -> [w686] mode=indexing
                    tunnel: [w684] -> w592 mode=indexing
                    tunnel: w621 -> [w685]
                    tunnel: [w685] -> w620
                    n139 = Index Array(array=w686, index=1) -> (element=w684:string)
                  }
                  n140 = call "WS1050 16 DUT AD7747 READ.vi"("error in"=w620, "Log (T)"=w612, "DUT Mask Mode (All)"=WSVCAP_SHL_I2C_DUT_Mask_Mode_Enum."C2") -> ("error out"=w618:errorcluster, "AD7747 Values"=w617:string[][])  [unwired: 7 in]
                  n141 = for {
                    tunnel: w617 -> [w682] mode=indexing
                    tunnel: [w680] -> w593 mode=indexing
                    tunnel: w618 -> [w681]
                    tunnel: [w681] -> w616
                    n142 = Index Array(array=w682, index=3) -> (element=w680:string)
                  }
                  n143 = call "WS1050 16 DUT AD7747 READ.vi"("error in"=w616, "Log (T)"=w612, "DUT Mask Mode (All)"=WSVCAP_SHL_I2C_DUT_Mask_Mode_Enum."C3") -> ("error out"=w614:errorcluster, "AD7747 Values"=w613:string[][])  [unwired: 7 in]
                  n144 = for {
                    tunnel: w613 -> [w678] mode=indexing
                    tunnel: [w676] -> w610 mode=indexing
                    tunnel: w614 -> [w677]
                    tunnel: [w677] -> w611
                    n145 = Index Array(array=w678, index=5) -> (element=w676:string)
                  }
                  n146 = case shown="0" w572 {
                    tunnel: w611 -> [w668 w675]
                    tunnel: [w668 w675] -> w587
                    tunnel: w610 -> [w665 w672]
                    tunnel: w593 -> [w666 w673]
                    tunnel: w592 -> [w667 w674]
                    tunnel: [w667 w674] -> w605
                    tunnel: [w666 w673] -> w606
                    tunnel: [w665 w672] -> w607
                    tunnel: [w665 w671] -> w590
                    tunnel: [w666 w670] -> w589
                    tunnel: [w667 w669] -> w588
                    frame 0 {
                      "C3 Min_T0" <- w665
                      "C2 Min_T0" <- w666
                      "C1 Min_T0" <- w667
                    }
                    frame 1, Default {
                      n147 = local read "C3 Min_T0"() -> (w671:string[])
                      n148 = local read "C1 Min_T0"() -> (w669:string[])
                      n149 = local read "C2 Min_T0"() -> (w670:string[])
                    }
                  }
                  n150 = Build Array(w592, w593, w610) -> (w594:string[][])
                  n151 = Transpose 2D Array(2D array=w594) -> (transposed array=→"CAP_Value(pF)":string[][])
                  n152 = call "WS1050 VSA_Delta C Calculation.vi"("error in (no error)"=w587, "CAP_T"=w605, "CAP_T0"=w588) -> ("error out"=w586:errorcluster, 2:"Delta C(pF)"=w596:dbl[], 3:"Delta C(pF)"=w604:string[])  [unwired: 6 in]
                  n153 = call "WS1050 VSA_Delta C Calculation.vi"("error in (no error)"=w587, "CAP_T"=w606, "CAP_T0"=w589) -> ("error out"=w585:errorcluster, 2:"Delta C(pF)"=w597:dbl[], 3:"Delta C(pF)"=w603:string[])  [unwired: 6 in]
                  n154 = call "WS1050 VSA_Delta C Calculation.vi"("error in (no error)"=w587, "CAP_T"=w607, "CAP_T0"=w590) -> ("error out"=w584:errorcluster, 2:"Delta C(pF)"=w598:dbl[], 3:"Delta C(pF)"=w602:string[])  [unwired: 6 in]
                }
                frame #1 {
                  n155 = Get Date/Time In Seconds() -> (seconds since 1Jan1904=w705:timestamp)
                  n156 = Concatenate Strings(w695, w708) -> (w707:string)
                  n157 = Get Date/Time String(seconds (now)=w705, want seconds? (F)=TRUE) -> (date string=→"date string":string, time string=→"Previous Time":string)  [unwired: 1 in]
                  n158 = Merge Errors(w699, w700, w698) -> (w697:errorcluster)
                  n159 = call "WS1050_16 DUT VSA Save Data Ver1.0.vi"("TMN DC\\CAP Data Log File Path"=w717, "Lot#"=w716, "VSA_Delta C1(pF)"=w711, "Wafer#"=w715, "File Name"=w712, "VSA_Delta C2(pF)"=w710, "error in"=w697, "Comment"=w707, "CP Current(uA)"=w713, "VSA_IDD(A)"="NA", "HD Time(Min)"=w688, "Driver"=w695, "VSA_C1"=w720, "CP HD (V)"=w694, "VSA_C2"=w719, "SN"=w714, "VSA_C3"=w718, "Test Program"=w693, "Voltage(V)"=w706, "Stress Voltage(V)"=w692, "VSA_Delta C3(pF)"=w709) -> ("error out"=w724:errorcluster)  [unwired: 6 in]
                }
              }
              n160 = Increment(x=w509) -> (x+1=→"Running Loops":i32)
              n161 = Build Array (concatenate)(w514, w517) -> (w513:dbl[])
              n162 = case shown="1, Default" w505 {
                tunnel: w508 -> [w567 w571]
                tunnel: w507 -> [w566 w570]
                tunnel: w506 -> [w565 w569]
                frame 0 {
                  n163 = Build Array(w567, w566, w565) -> (→"Delta CAP_T0(pF)":dbl[][])
                }
                frame 1, Default {
                  n164 = Build Array(w571, w570, w569) -> (→"Delta CAP_Tc(pF)":dbl[][])
                }
              }
              n165 = call "Delay T4.vi"("milliseconds to wait"=u32 10, "error in (no error)"=w558) -> ("error out"=w561:errorcluster)  [unwired: 9 in]
              n166 = Unbundle By Name(w561) -> ("status"=w536:bool)
              n167 = Compound Arithmetic op=OR(w536, w526) -> (w525:bool)
            }
            n168 = Unbundle By Name(w458) -> ("status"=w475:bool)
            n169 = Or(x=w475, y=w474) -> (x .or. y?=w473:bool)
            n170 = call "Delay T4.vi"("milliseconds to wait"=u32 10, "error in (no error)"=w458) -> ("error out"=w471:errorcluster)  [unwired: 9 in]
          }
          n171 = flat-sequence {
            tunnel: w297 -> [w340]
            tunnel: [w340] -> w296
            tunnel: w294 -> [w338]
            tunnel: [w339] -> w295
            frame #0 {
              n172 = Greater Or Equal?(x=w338, y="Set HD Time \nto Complete(Min)") -> (x >= y?=w339:bool)
              "HD Time\nCompleted(Min)" <- w338
            }
          }
          n173 = Unbundle By Name(w296) -> ("status"=w299:bool)
          n174 = call "Delay T4.vi"("milliseconds to wait"=u32 50, "error in (no error)"=w296) -> ("error out"=w311:errorcluster)  [unwired: 9 in]
          n175 = Compound Arithmetic op=OR(w295, w299, w289) -> (w267:bool)
        }
        n176 = VISA Write(VISA resource name=w241, write buffer="SOUR:FUNC VOLT;VOLT:MODE FIX;RANG 100;LEV 0.0;:SENS:FUNC \"CURR\";CURR:PROT 60E-3;RANG 100E-3;:OUTP ON", error in (no error)=w232) -> (VISA resource name out=w245:refnum<visa-resource-name>, error out=w236:errorcluster)  [unwired: 1 out]
        n177 = for {
          tunnel: w235 -> [w259]
          tunnel: w237 -> [w256] mode=indexing
          shift-right: [w254] -> w231
          shift-left: w236 -> [w260]
          tunnel: [w252] -> w234
          n178 = call "E3631A_Voltage Controller updated.vi"("VISA resource name"=w259, "I_VDD(A)"=0.2, "Channel Controller"=w256, "Voltage 1"=0.0, "Voltage 2"=3.3, "error in (no error)"=w260, "Voltage 3"=-3.3) -> ("VISA resource name out"=w252:refnum<visa-resource-name>, "error out"=w255:errorcluster)  [unwired: 7 in]
          n179 = call "Delay T4.vi"("milliseconds to wait"=u32 100, "error in (no error)"=w255) -> ("error out"=w254:errorcluster)  [unwired: 9 in]
        }
        n180 = flat-sequence {
          tunnel: w231 -> [w727]
          tunnel: [w727] -> w230
          frame #0 {
            n181 = local write "STATUS"("Idle...." ("STATUS")) -> ()
            n182 = One Button Dialog(message="Test Completed") -> ()  [unwired: 1 in, 1 out]
          }
        }
      }
      frame True {
        w730 = FALSE
      }
    }
    n183 = Wait Until Next ms Multiple(millisecond multiple=u32 100) -> ()  [unwired: 1 out]
    n184 = local write "Abort"(w54) -> ()
    n185 = local write "stop"(w55) -> ()
    n186 = Unbundle By Name(w57) -> ("status"=w73:bool)
    n187 = Compound Arithmetic op=OR(w50, w73, w65) -> (w72:bool)
  }
  "Ke2000 Out" <- w24
  "PS1 Out" <- w23
  n188 = local write "Abort"(w8) -> ()
  n189 = local write "stop"(w8) -> ()
  n190 = case shown="True" w21 {
    tunnel: [w735 w737] -> w7
    tunnel: w15 -> [w735 w736]
    frame False {
    }
    frame True {
      n191 = flat-sequence {
        tunnel: w736 -> [w740]
        tunnel: [w739] -> w737
        frame #0 {
          n192 = local write "Online"(FALSE ("Online")) -> ()
          n193 = call "WSVCAP SHL Host TL Close.vi"("error in"=w740) -> ("error out"=w739:errorcluster)  [unwired: 14 in]
        }
      }
    }
  }
  "error out" <- w7
  n194 = VISA Write(VISA resource name=w16, write buffer="SOUR:FUNC VOLT;VOLT:MODE FIX;RANG 100;LEV 0.0;:SENS:FUNC \"CURR\";CURR:PROT 60E-3;RANG 100E-3;:OUTP OFF", error in (no error)=w15) -> (VISA resource name out=→"VISA resource name out":refnum<visa-resource-name>, error out=→"error out 2":errorcluster)  [unwired: 1 out]
